vi "Save_to_JSON.vi"() -> ()   [LabVIEW 2019]
uses:
  c3a6e8a8-a6df-4c09-aa6b-e6661d54ffd0.vi
  <vilib>/JDP Science/JSONtext/Variant to JSON Text.vi
  <vilib>/JDP Science/JSONtext/JSONtext.lvlib
panel:
  in  "Samples per freq calc":dbl=10000.0
  in  "Folder":path
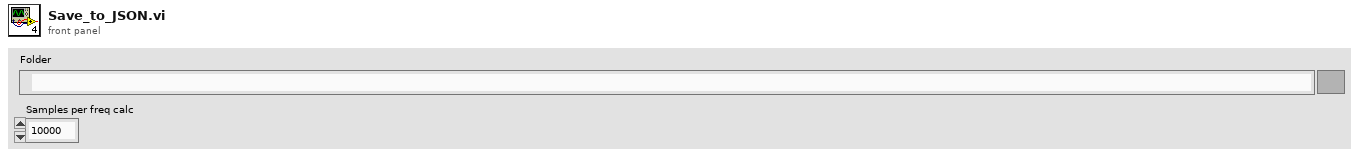
[diagram p1: front panel]
types:
  T1 = enum16{"open", "replace", "create", "open or create", "replace or create", "replace or create with confirmation"}
  T2 = enum16{"open", "open or create", "create or replace", "create", "open (read-only)"}
  T3 = cluster{"x":dbl[], "y":dbl[], "z":dbl[], "rpm":dbl[], "t":dbl[]}
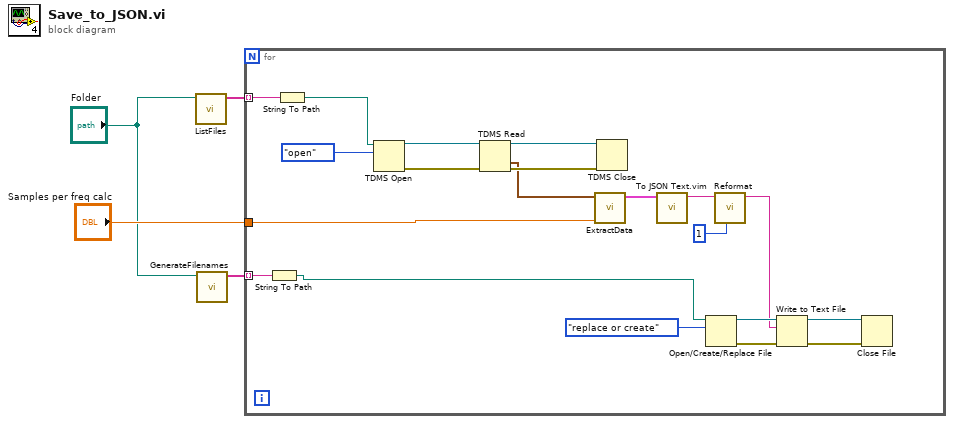
[diagram p0: block diagram]
diagram:
  n1 = call "ListFiles.vi"("Folder"="Folder") -> ("TDMS"=w3:string[])  [unwired: 10 in]
  n2 = call "GenerateFilenames.vi"("Path"="Folder") -> ("Array"=w2:string[])  [unwired: 10 in]
  n3 = for {
    tunnel: "Samples per freq calc" -> [w18]
    tunnel: w3 -> [w8] mode=indexing
    tunnel: w2 -> [w6] mode=indexing
    n4 = String To Path(string=w6) -> (path=w5:path)
    n5 = String To Path(string=w8) -> (path=w7:path)
    n6 = TDMS Open(10:T2."open" ("operation (0:open)"), 11:w7) -> (0:w22:errorcluster, 3:w23:refnum<k34>)  [unwired: 5 in]
    n7 = TDMS Read(0:w23, 11:w22) -> (4:w21:refnum<k34>, 10:w19:waveform(dbl)[], 15:w20:errorcluster)  [unwired: 6 in, 3 out]
    n8 = call "ExtractData.vi"("Samples per freq calc"=w18, "Data input"=w19) -> ("Data cluster"=w12:T3)  [unwired: 9 in]
    n9 = TDMS Close(8:w20, 11:w21) -> ()  [unwired: 2 out]
    n10 = call "To JSON Text.vim"("Anything"=w12) -> ("<JSON>"=w11:string)  [unwired: 9 in, 1 out]
    n11 = Open/Create/Replace File(file path (use dialog)=w5, operation (0:open)=T1."replace or create") -> (refnum out=w15:refnum<file>, error out=w14:errorcluster)  [unwired: 4 in, 1 out]
    n12 = call <vilib>:"Reformat.vi"("Pretty Print Levels"=1, "JSON"=w11) -> ("<JSON>First JSON Value\n\n<JSON>"=w10:string)  [unwired: 6 in, 3 out]
    n13 = Write to Text File(file (use dialog)=w15, text=w10, error in=w14) -> (refnum out=w17:refnum<file>, error out=w16:errorcluster)  [unwired: 1 in, 1 out]
    n14 = Close File(refnum=w17, error in=w16) -> ()  [unwired: 2 out]
  }
